vi "rxCRC.vi"(8 "error in":errorcluster, 10 "inputData":dbl[](array[numeric]), 11 "Path In":path) -> (0 "error out":errorcluster, 1 "out_data":dbl[](array[numeric]), 2 "CRC_flag":dbl, 3 "Path Out":path)   [LabVIEW 2015]
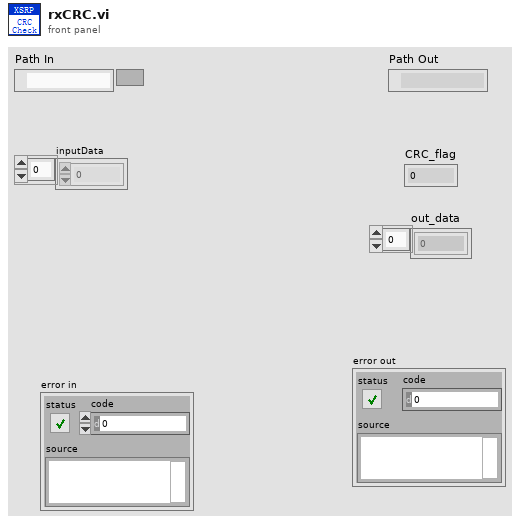
[diagram p1: front panel]
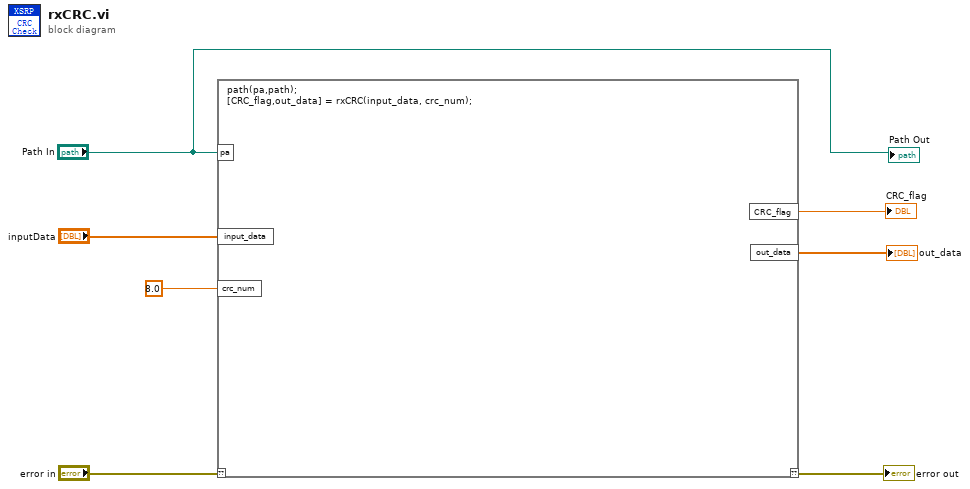
[diagram p0: block diagram]
diagram:
  n1 = script code="path(pa,path);\n[CRC_flag,out_data] = rxCRC(input_data, crc_num);"("??"="error in", "pa"="Path In", "input_data"="inputData", "crc_num"=8.0) -> ("??"=→"error out":errorcluster, "CRC_flag"=→"CRC_flag":dbl, "out_data"=→"out_data":dbl[])
  "Path Out" <- "Path In"
